vi "Input Var.vi"() -> ()   [LabVIEW 2016, in "EXO2-Sonde.lvlib"]
uses:
  EXO2-Sonde.lvlib
panel:
  out "EXO message":T1
  out "EXO原始数据包":string
  out "收到监测数据":bool
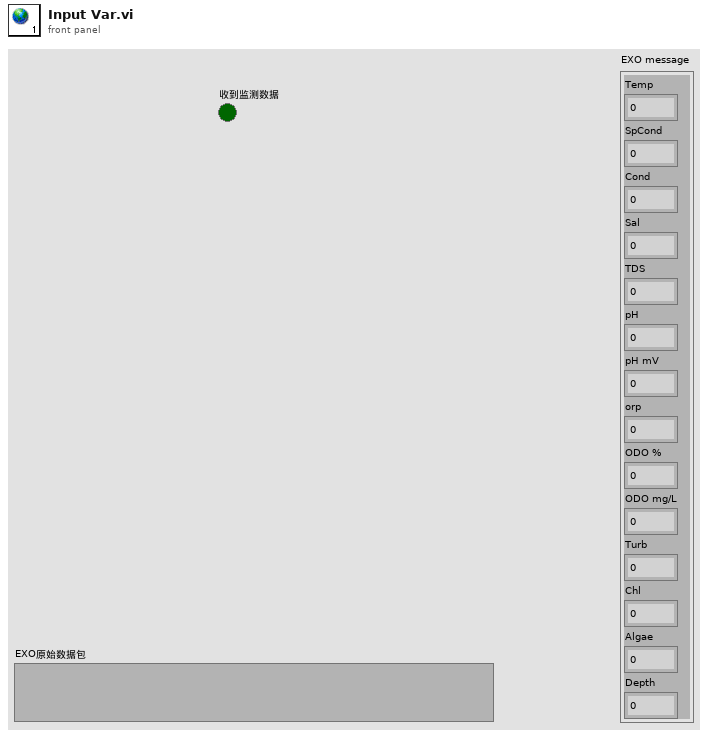
[diagram p1: front panel]
types:
  T1 = cluster{"Temp":dbl, "SpCond":dbl, "Cond":dbl, "Sal":dbl, "TDS":dbl, "pH":dbl, "pH mV":dbl, "orp":dbl, "ODO %":dbl, "ODO mg/L":dbl, "Turb":dbl, "Chl":dbl, "Algae":dbl, "Depth":dbl}
diagram:
